vi "rmad regobs api.vi"(4 "Id":string="c4fc2c1e-040f-42cb-9744-3138bbf46919", 5 "RegId":i32=103004, 6 "base url":string="https://tst-h-web03.nve.no/regobswebapi/", 7 "State":u16(ring)=1 items=["Insert new observation", "Get observation"], 8 "error in (no error)":errorcluster, 9 "DtObsTime":string="2018-01-01T00:00:00.000Z", 10 "ObsLocation":cluster{"ObsLocationId":i32}={"ObsLocationId"=62943} {"ObsLocationId" items=["Lauvjuvet"=66553, "Sandneslia"=66555, "Lauvjuvet Demo"=47721, "Sandneslia Demo"=47724, "Lauvjuvet Test"=62943, "Sandneslia Test"=62942, "F46 test"=63942]}, 11 "AvalancheObs":T1={"DtAvalancheTime"="2018-01-01T00:00:00.000Z", "DestructiveSizeTID"=2, "AvalancheTriggerTID"=10, "AvalancheTID"=12, "TerrainStartZoneTID"=40, "ValidExposition"="00000100", "Trajectory"="Lauvjuvet", "StartLat"=59.76323320145381, "StartLong"=7.813512796395109, "StopLat"=59.75649048544803, "StopLong"=7.808107516195507, "Comment"="Automatisk skredvarsling med goefoner"} {"DestructiveSizeTID" items=["Ikke gitt"=0, "1-Harmløs"=1, "2-Små"=2, "3-Middels"=3, "4-Stort"=4, "5-Svært stort"=5, "Ukjent"=9]; "AvalancheTriggerTID" items=["Ikke gitt"=0, "Naturlig utløst"=10, "Kunstig utløst"=20, "Ski eller skuter utløst"=21, "Ski eller skuter fjernutløst"=22, "Kunstig utløst testheng"=23, "Utløst med sprengstoff"=25, "Ukjent"=99]; "AvalancheTID" items=["Ikke gitt"=0, "Tørt løssnøskred"=12, "Vått løssnøskred"=11, "Tørt flakskred"=22, "Vått flakskred"=21, "Glideskred"=27, "Sørpeskred"=30, "Skavlfall"=40, "Ukjent"=99]; "TerrainStartZoneTID" items=["Ikke gitt"=0, "Brattheng"=10, "Leområder"=20, "Nær rygg"=30, "I renne eller forsenkning"=40, "Svaberg"=50, "Skål"=60, "I skogen"=70, "Hogstfelt"=75, "Overalt i terrenget"=95, "Ukjent"=99]}) -> (0 "error out":errorcluster, 1 "body insert":string, 3 "value":T2 {"Results"."Registrations"."FullObject"."StartPoint"."Latitude" format="%.8g"; "Results"."Registrations"."FullObject"."StartPoint"."Longitude" format="%.8g"; "Results"."Registrations"."FullObject"."StopPoint"."Latitude" format="%.8g"; "Results"."Registrations"."FullObject"."StopPoint"."Longitude" format="%.8g"})   [LabVIEW 2017]
uses:
  <vilib>/httpClient/POSTBuffer.vi
  <vilib>/httpClient/LabVIEWHTTPClient.lvlib
panel:
  out "concatenated string 2":string
  out "concatenated string":string
  out "Insert observation JSON string":string
  out "headers  insert":string
  out "headers  get":string
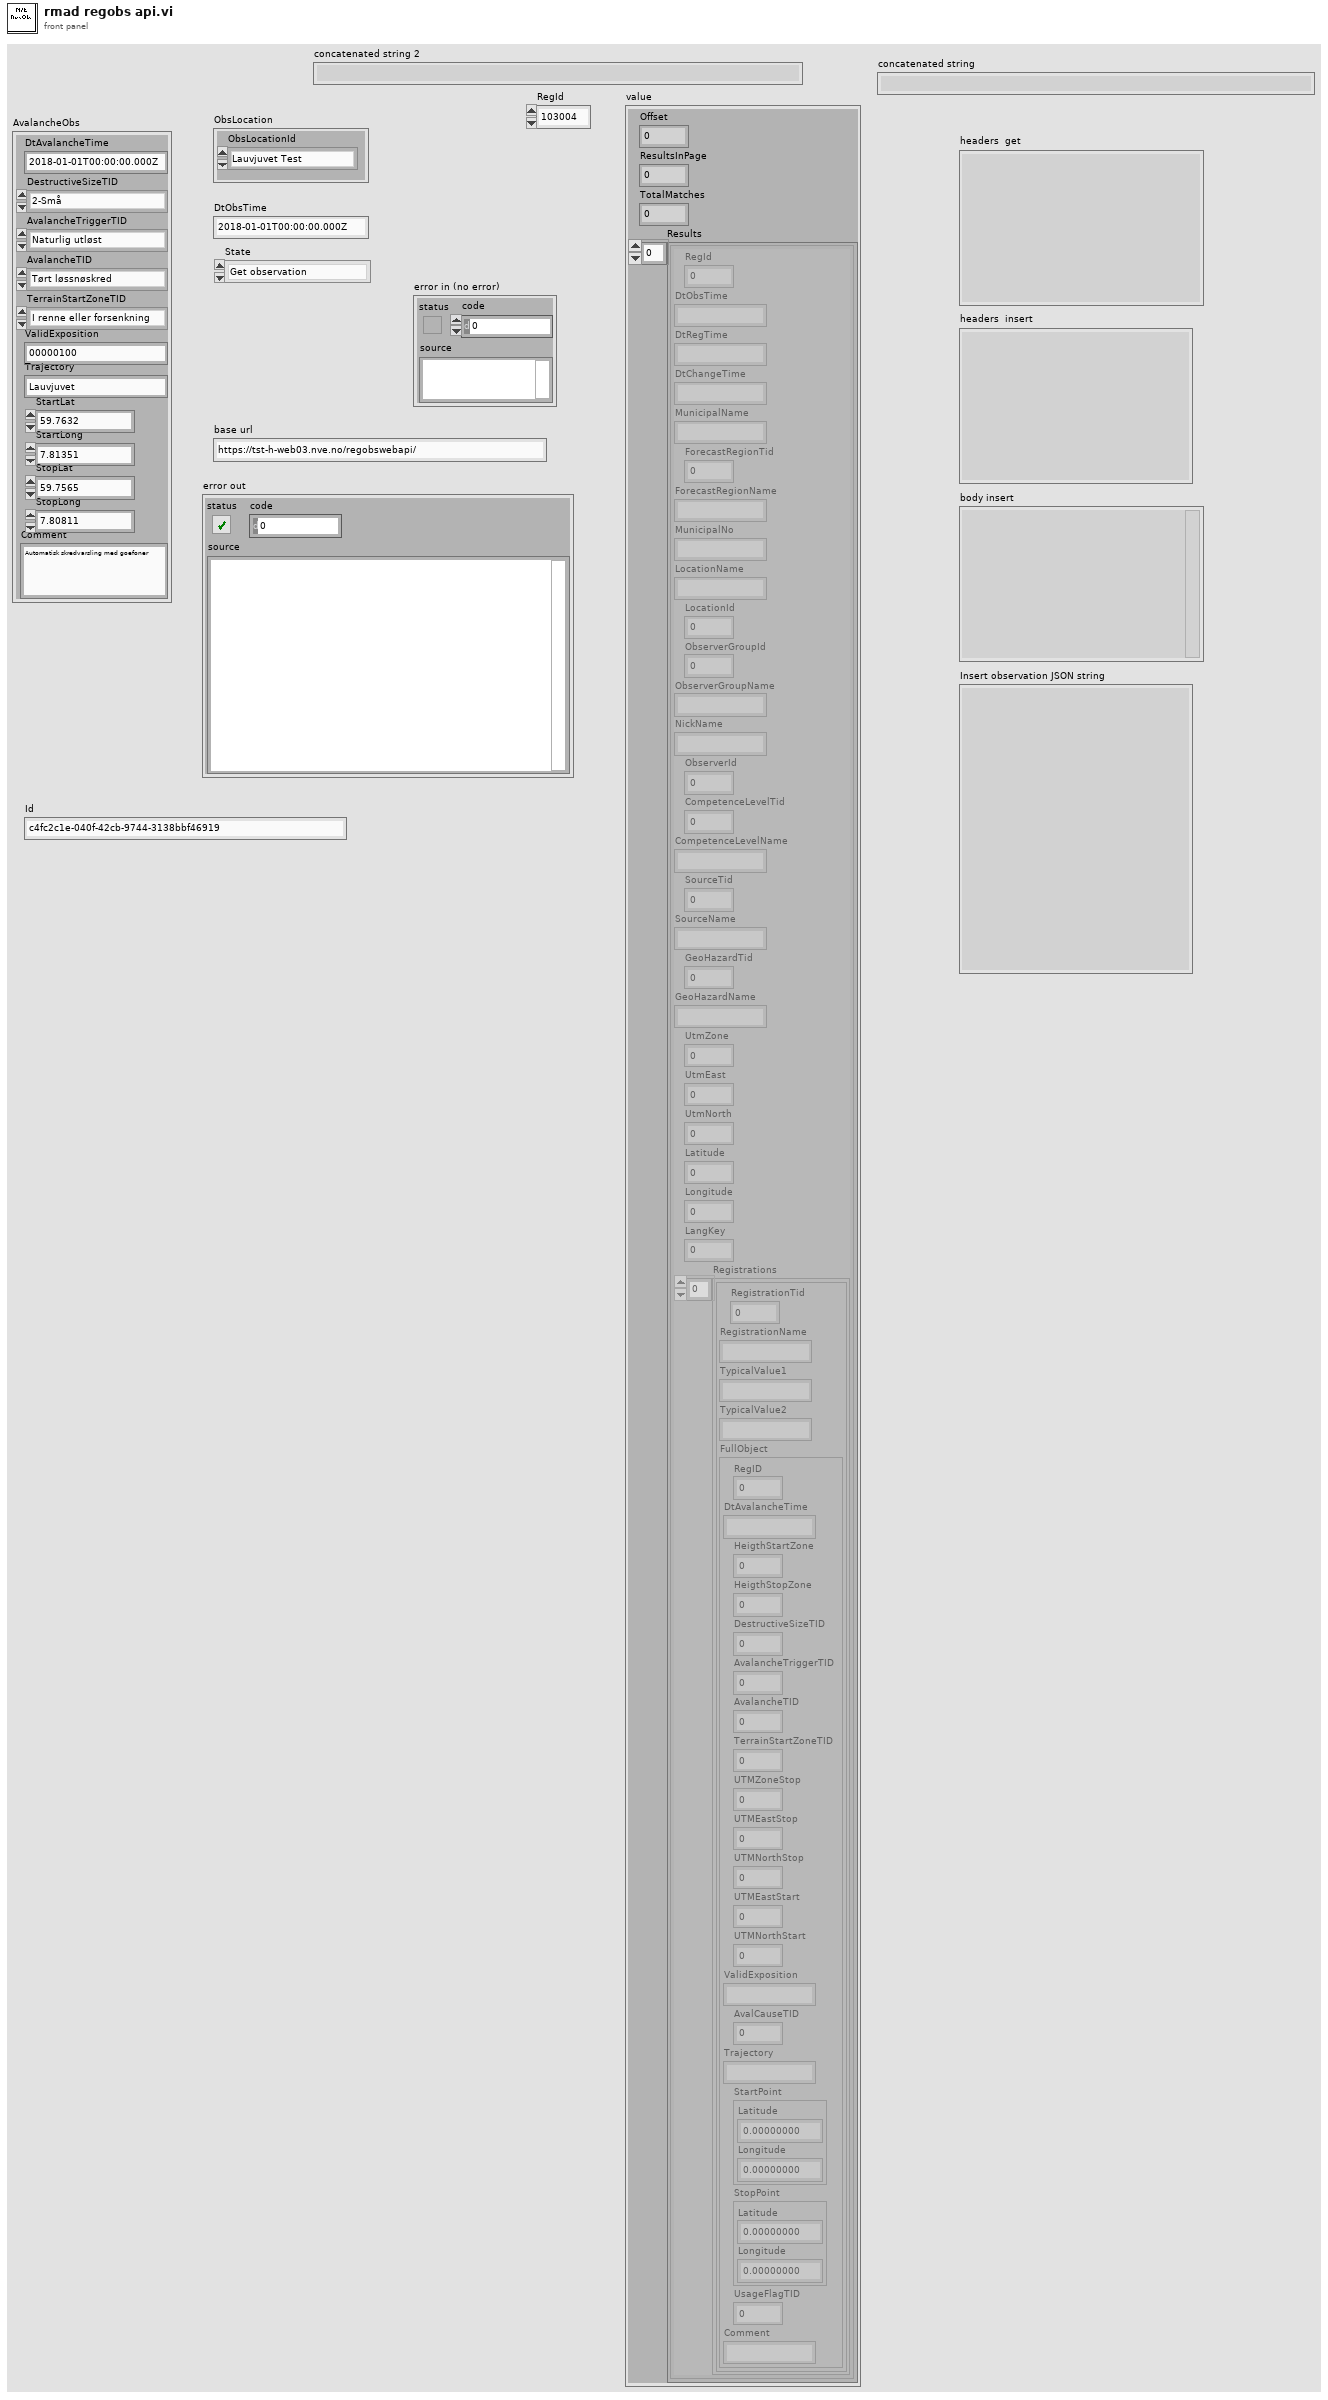
[diagram p1: front panel]
types:
  T1 = cluster{"DtAvalancheTime":string, "DestructiveSizeTID":i32, "AvalancheTriggerTID":i32, "AvalancheTID":i32, "TerrainStartZoneTID":i32, "ValidExposition":string, "Trajectory":string, "StartLat":dbl, "StartLong":dbl, "StopLat":dbl, "StopLong":dbl, "Comment":string}
  T2 = cluster{"Offset":i32, "ResultsInPage":i32, "TotalMatches":i32, "Results":cluster{"RegId":i32, "DtObsTime":string, "DtRegTime":string, "DtChangeTime":string, "MunicipalName":string, "ForecastRegionTid":i32, "ForecastRegionName":string, "MunicipalNo":string, "LocationName":string, "LocationId":i32, "ObserverGroupId":i32, "ObserverGroupName":string, "NickName":string, "ObserverId":i32, "CompetenceLevelTid":i32, "CompetenceLevelName":string, "SourceTid":i32, "SourceName":string, "GeoHazardTid":i32, "GeoHazardName":string, "UtmZone":i32, "UtmEast":i32, "UtmNorth":i32, "Latitude":dbl, "Longitude":dbl, "LangKey":i32, "Registrations":cluster{"RegistrationTid":i32, "RegistrationName":string, "TypicalValue1":string, "TypicalValue2":string, "FullObject":cluster{"RegID":i32, "DtAvalancheTime":string, "HeigthStartZone":i32, "HeigthStopZone":i32, "DestructiveSizeTID":i32, "AvalancheTriggerTID":i32, "AvalancheTID":i32, "TerrainStartZoneTID":i32, "UTMZoneStop":i32, "UTMEastStop":i32, "UTMNorthStop":i32, "UTMEastStart":i32, "UTMNorthStart":i32, "ValidExposition":string, "AvalCauseTID":i32, "Trajectory":string, "StartPoint":cluster{"Latitude":dbl, "Longitude":dbl}, "StopPoint":cluster{"Latitude":dbl, "Longitude":dbl}, "UsageFlagTID":i32, "Comment":string}}[]}[]}
  T3 = cluster{"Latitude":string, "Longitude":string, "Uncertainty":string, "UTMSourceTID":string}
  T4 = cluster{"DtAvalancheTime":string, "HightStartZone":string, "HightStopZone":string, "DestructiveSizeTID":i32, "AvalancheTriggerTID":i32, "AvalancheTID":i32, "TerrainStartZoneTID":i32, "UTMZoneStop":i32, "UTMEastStop":i32, "UTMNorthStop":i32, "UTMEastStart":i32, "UTMNorthStart":i32, "ValidExposition":string, "AvalCauseTID":i32, "Trajectory":string, "StartLat":dbl, "StartLong":dbl, "StopLat":dbl, "StopLong":dbl, "UsageFlagTID":i32, "Comment":string}
  T5 = cluster{"RegId":i32, "DtObsTime":string, "DtRegTime":string, "DtChangeTime":string, "MunicipalName":string, "ForecastRegionTid":i32, "ForecastRegionName":string, "MunicipalNo":string, "LocationName":string, "LocationId":i32, "ObserverGroupId":i32, "ObserverGroupName":string, "NickName":string, "ObserverId":i32, "CompetenceLevelTid":i32, "CompetenceLevelName":string, "SourceTid":i32, "SourceName":string, "GeoHazardTid":i32, "GeoHazardName":string, "UtmZone":i32, "UtmEast":i32, "UtmNorth":i32, "Latitude":dbl, "Longitude":dbl, "LangKey":i32, "Registrations":cluster{"RegistrationTid":i32, "RegistrationName":string, "TypicalValue1":string, "TypicalValue2":string, "FullObject":cluster{"RegID":i32, "DtAvalancheTime":string, "HeigthStartZone":i32, "HeigthStopZone":i32, "DestructiveSizeTID":i32, "AvalancheTriggerTID":i32, "AvalancheTID":i32, "TerrainStartZoneTID":i32, "UTMZoneStop":i32, "UTMEastStop":i32, "UTMNorthStop":i32, "UTMEastStart":i32, "UTMNorthStart":i32, "ValidExposition":string, "AvalCauseTID":i32, "Trajectory":string, "StartPoint":cluster{"Latitude":dbl, "Longitude":dbl}, "StopPoint":cluster{"Latitude":dbl, "Longitude":dbl}, "UsageFlagTID":i32, "Comment":string}}[]}[]
  T6 = typedef "LabVIEWHTTPClient.lvlib/ClientHandle.ctl" = refnum<k1>
  T7 = cluster{"Id":string, "ObserverGroupID":i32, "GeoHazardTID":i32, "ObserverGuid":string, "DtObsTime":string, "ObsLocation":cluster{"ObsLocationId":i32}, "AvalancheObs":cluster{"DtAvalancheTime":string, "DestructiveSizeTID":i32, "AvalancheTriggerTID":i32, "AvalancheTID":i32, "TerrainStartZoneTID":i32, "ValidExposition":string, "Trajectory":string, "StartLat":dbl, "StartLong":dbl, "StopLat":dbl, "StopLong":dbl, "Comment":string}}
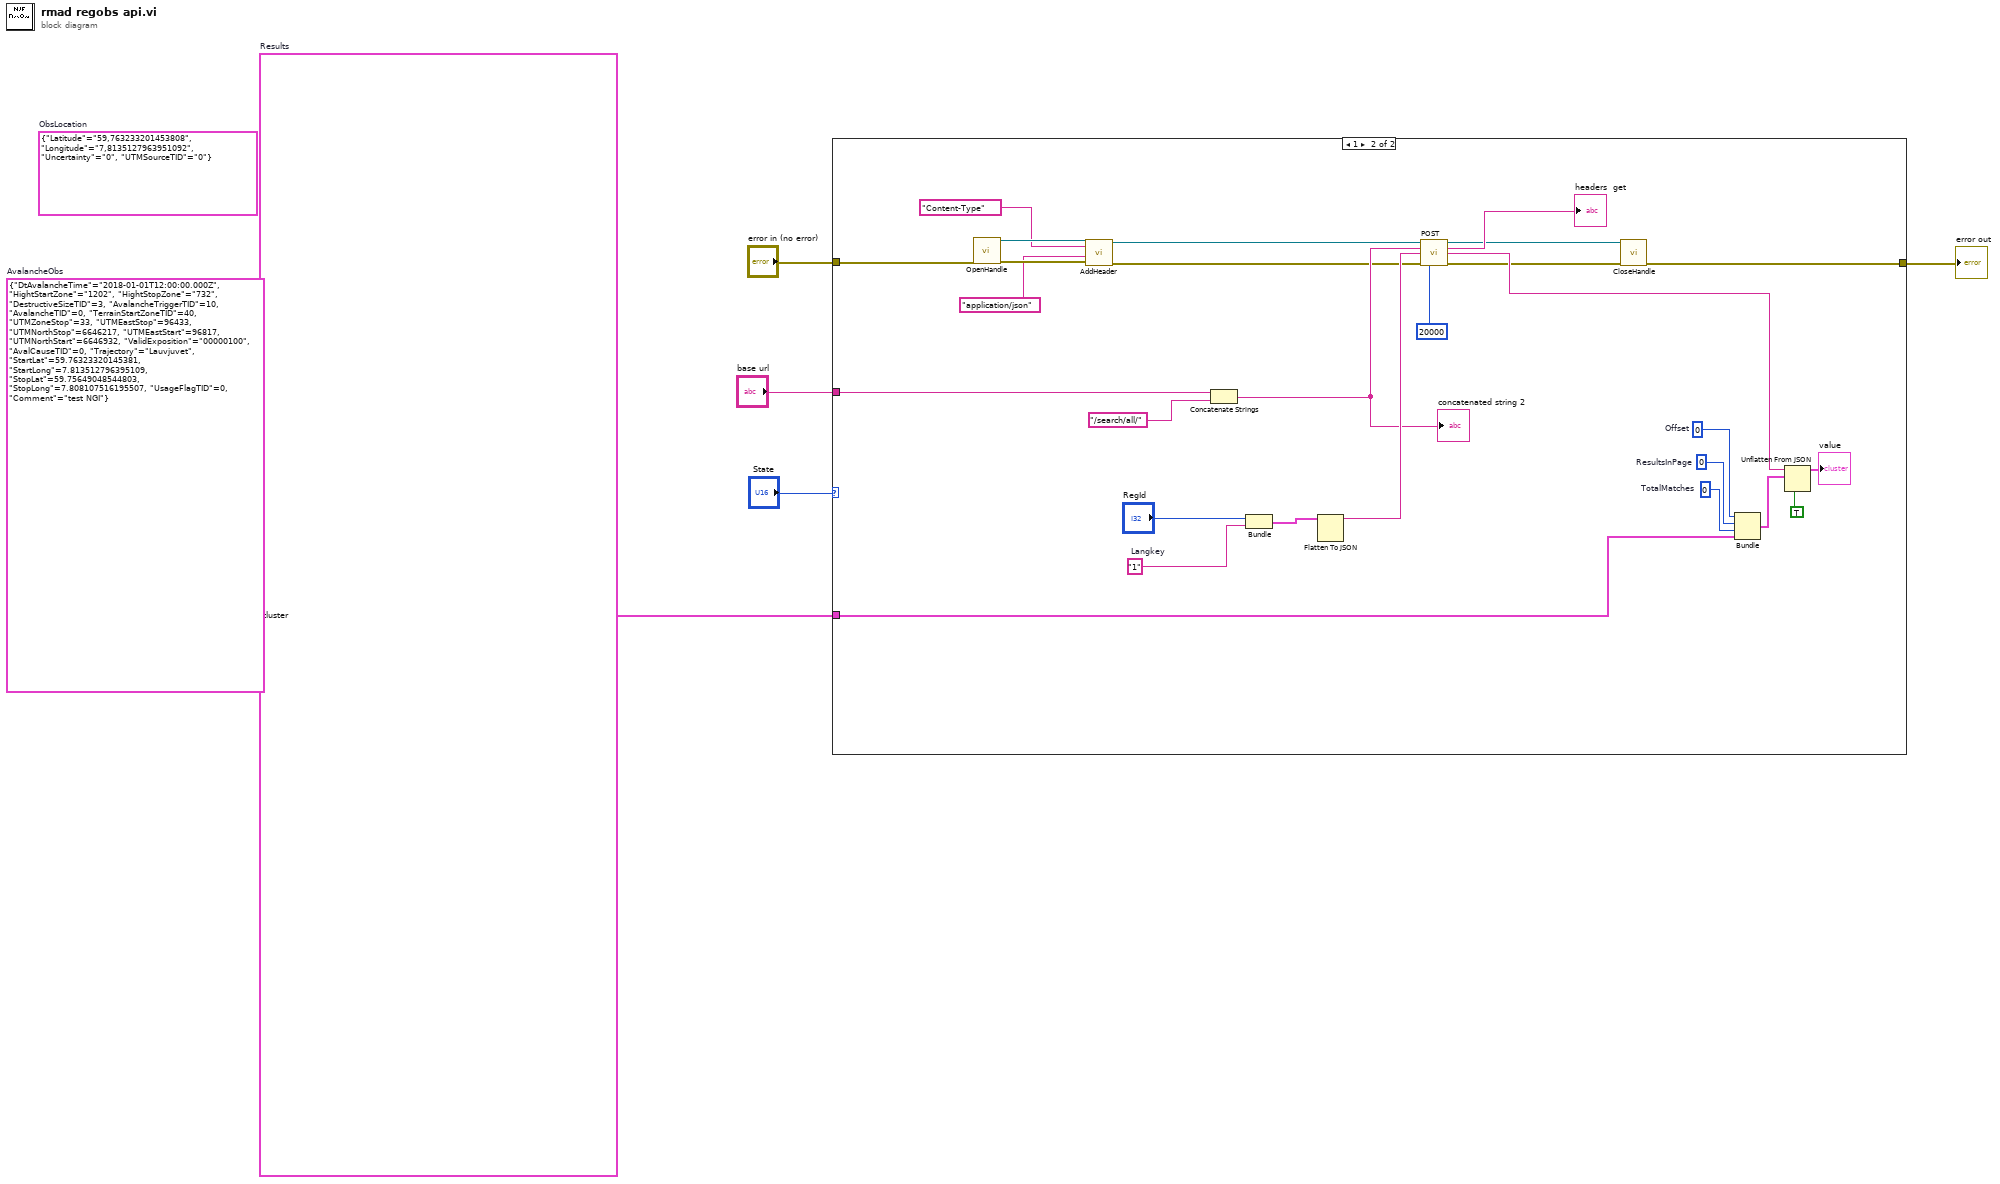
[diagram p0: block diagram]
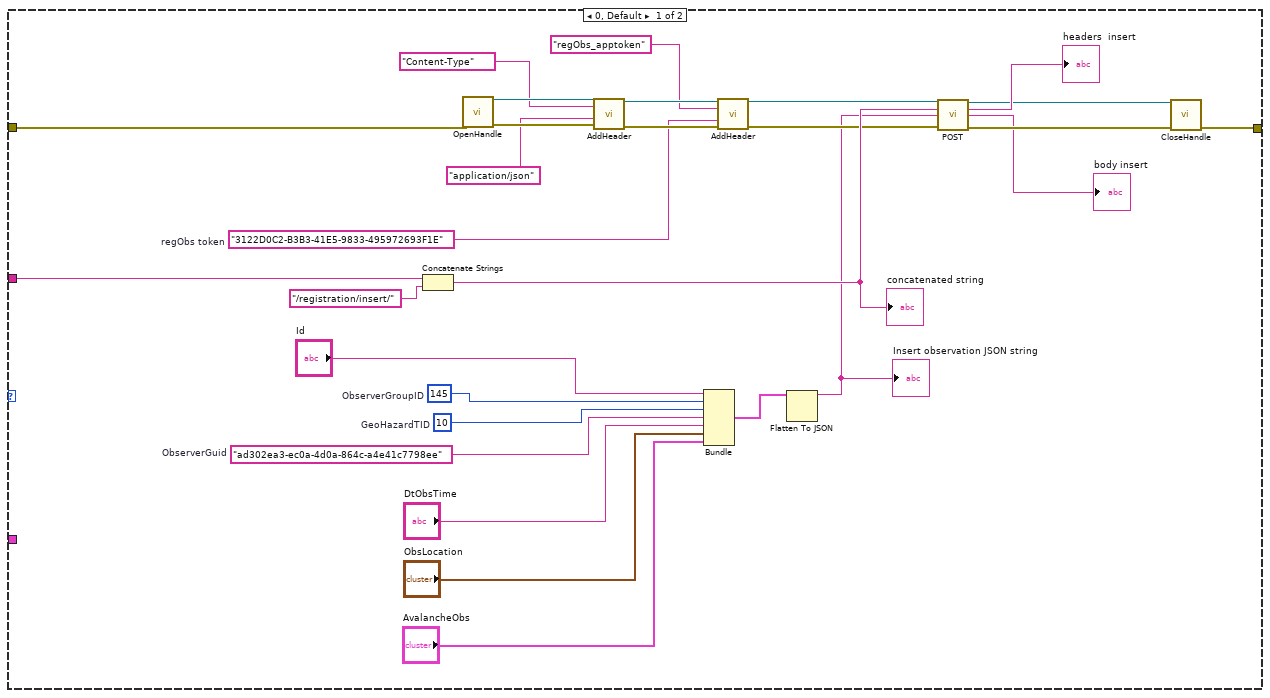
[diagram p2: hidden frame]
diagram:
  (unwired) T3 {"Latitude"="59,763233201453808", "Longitude"="7,8135127963951092", "Uncertainty"="0", "UTMSourceTID"="0"}  # ObsLocation
  (unwired) T4 {"DtAvalancheTime"="2018-01-01T12:00:00.000Z", "HightStartZone"="1202", "HightStopZone"="732", "DestructiveSizeTID"=3, "AvalancheTriggerTID"=10, "AvalancheTID"=0, "TerrainStartZoneTID"=40, "UTMZoneStop"=33, "UTMEastStop"=96433, "UTMNorthStop"=6646217, "UTMEastStart"=96817, "UTMNorthStart"=6646932, "ValidExposition"="00000100", "AvalCauseTID"=0, "Trajectory"="Lauvjuvet", "StartLat"=59.76323320145381, "StartLong"=7.813512796395109, "StopLat"=59.75649048544803, "StopLong"=7.808107516195507, "UsageFlagTID"=0, "Comment"="test NGI"}  # AvalancheObs
  w2 = T5 [{"RegId"=0, "DtObsTime"="", "DtRegTime"="", "DtChangeTime"="", "MunicipalName"="", "ForecastRegionTid"=0, "ForecastRegionName"="", "MunicipalNo"="", "LocationName"="", "LocationId"=0, "ObserverGroupId"=0, "ObserverGroupName"="", "NickName"="", "ObserverId"=0, "CompetenceLevelTid"=0, "CompetenceLevelName"="", "SourceTid"=0, "SourceName"="", "GeoHazardTid"=0, "GeoHazardName"="", "UtmZone"=0, "UtmEast"=0, "UtmNorth"=0, "Latitude"=0.0, "Longitude"=0.0, "LangKey"=0, "Registrations"=[{"RegistrationTid"=0, "RegistrationName"="", "TypicalValue1"="", "TypicalValue2"="", "FullObject"={"RegID"=0, "DtAvalancheTime"="2018-01-01T12:00:00.000Z", "HeigthStartZone"=0, "HeigthStopZone"=0, "DestructiveSizeTID"=3, "AvalancheTriggerTID"=10, "AvalancheTID"=0, "TerrainStartZoneTID"=40, "UTMZoneStop"=33, "UTMEastStop"=96433, "UTMNorthStop"=6646217, "UTMEastStart"=96817, "UTMNorthStart"=6646932, "ValidExposition"="00000100", "AvalCauseTID"=0, "Trajectory"="Lauvjuvet", "StartPoint"={"Latitude"=59.76323320145381, "Longitude"=7.813512796395109}, "StopPoint"={"Latitude"=59.75649048544803, "Longitude"=7.808107516195507}, "UsageFlagTID"=0, "Comment"="test NGI"}}]}]  # Results
  n1 = case shown="1" "State" {
    tunnel: [w12 w46] -> w1
    tunnel: "error in (no error)" -> [w26 w45]
    tunnel: "base url" -> [w25 w44]
    tunnel: w2 -> [_ w37]
    frame 0, Default {
      w9 = 145  # ObserverGroupID
      w15 = 10  # GeoHazardTID
      w16 = "ad302ea3-ec0a-4d0a-864c-a4e41c7798ee"  # ObserverGuid
      w10 = "3122D0C2-B3B3-41E5-9833-495972693F1E"  # regObs token
      n2 = Concatenate Strings(w25, "/registration/insert/") -> (w24:string)
      "concatenated string" <- w24
      n3 = call <vilib>:"OpenHandle.vi"("error in (no error)"=w26) -> ("client handle out"=w31:T6, "error out"=w32:errorcluster)  [unwired: 13 in]
      n4 = call <vilib>:"AddHeader.vi"("client handle"=w31, "header"="Content-Type", "value"="application/json", "error in (no error)"=w32) -> ("client handle out"=w21:T6, "error out"=w22:errorcluster)  [unwired: 10 in]
      n5 = Bundle("Id"="Id", "ObserverGroupID"=w9, "GeoHazardTID"=w15, "ObserverGuid"=w16, "DtObsTime"="DtObsTime", "ObsLocation"="ObsLocation", "AvalancheObs"="AvalancheObs") -> (w13:T7)  [unwired: 1 in]
      n6 = call <vilib>:"AddHeader.vi"("client handle"=w21, "header"="regObs_apptoken", "value"=w10, "error in (no error)"=w22) -> ("client handle out"=w19:T6, "error out"=w20:errorcluster)  [unwired: 10 in]
      n7 = Flatten To JSON(anything=w13) -> (JSON string=w17:string)  [unwired: 2 in, 1 out]
      "Insert observation JSON string" <- w17
      n8 = call-poly <vilib>:"POST.vi"("client handle"=w19, "url"=w24, "buffer"=w17, "error in (no error)"=w20) -> ("client handle out"=w27:T6, "headers"=→"headers  insert":string, "body"=→"body insert":string, "error out"=w28:errorcluster)  [unwired: 8 in]
      n9 = call <vilib>:"CloseHandle.vi"("client handle"=w27, "error in (no error)"=w28) -> ("error out"=w12:errorcluster)  [unwired: 13 in]
    }
    frame 1 {
      w38 = "1"  # Langkey
      w56 = 0  # TotalMatches
      w58 = 0  # ResultsInPage
      w57 = 0  # Offset
      n10 = call <vilib>:"OpenHandle.vi"("error in (no error)"=w45) -> ("client handle out"=w52:T6, "error out"=w53:errorcluster)  [unwired: 13 in]
      n11 = call <vilib>:"AddHeader.vi"("client handle"=w52, "header"="Content-Type", "value"="application/json", "error in (no error)"=w53) -> ("client handle out"=w40:T6, "error out"=w39:errorcluster)  [unwired: 10 in]
      n12 = Concatenate Strings(w44, "/search/all/") -> (w43:string)
      "concatenated string 2" <- w43
      n13 = Bundle("RegId"="RegId", "Langkey"=w38) -> (w55:cluster{"RegId":i32, "Langkey":string})  [unwired: 1 in]
      n14 = Flatten To JSON(anything=w55) -> (JSON string=w48:string)  [unwired: 2 in, 1 out]
      n15 = call-poly <vilib>:"POST.vi"("client handle"=w40, "url"=w43, "buffer"=w48, "error in (no error)"=w39, "timeout (10000)"=20000) -> ("client handle out"=w47:T6, "headers"=→"headers  get":string, "body"=w59:string, "error out"=w49:errorcluster)  [unwired: 7 in]
      n16 = call <vilib>:"CloseHandle.vi"("client handle"=w47, "error in (no error)"=w49) -> ("error out"=w46:errorcluster)  [unwired: 13 in]
      n17 = Bundle("Offset"=w57, "ResultsInPage"=w58, "TotalMatches"=w56, "Results"=w37) -> (w41:T2)  [unwired: 1 in]
      n18 = Unflatten From JSON(JSON string=w59, type and defaults=w41, default null elements? (F)=TRUE) -> (value=→"value":T2)  [unwired: 4 in, 1 out]
    }
  }
  "error out" <- w1
